vi "JIO_OnePannel_ChannelSweep_Ken.vi"() -> ()   [LabVIEW 2023, in "JIO.lvlib"]
uses:
  JIO.lvlib
  CTL/Mode_tx1_rx2.ctl
  FTDI/JIO/CLC_JIO_FTDI.lvlib
  R_S/R_S.lvlib
  Anritsu/Anritsu.lvlib
panel:
  in  "Mode":T1=enum."Tx"
  in  "ud att":i32
  in  "AvgTimes":i32=1
  in  "SA":refnum<visa-resource-name>="TCPIP0::192.168.100.202::inst0::INSTR"
  in  "File_note":string
  out "error out":errorcluster
  out "Time(64-Steps)sec":dbl
  out "Phase":i32
  out "Channel":i32
  out "IC_No.":i32
  out "Chain":i32
  out "Spectrum":dbl[](graph)
  in  "Waiting Time(ms)":u32=1000
  in  "error in":errorcluster
  in  "Ref_gain":i32
  in  "Ref_Phase":i32
  in  "Ref_Channel":i32
  in  "Ref_IC_":i32
  in  "Ref_Chain":i32
  in  "Channel_setting":T2
  # "CLC Gen4 8x4 Channel Sweep for TMYTEK"
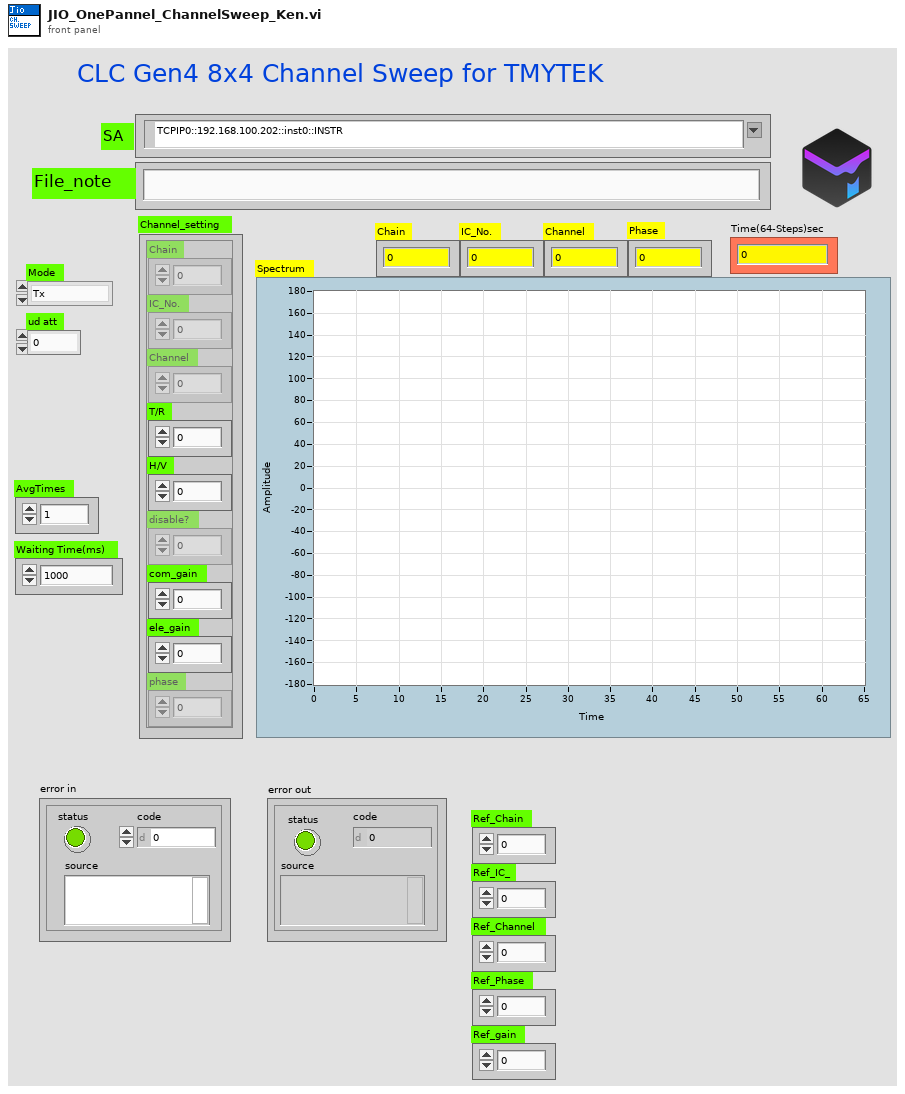
[diagram p1: front panel]
types:
  T1 = typedef "Mode_tx1_rx2.ctl" = enum16{"Standy", "Tx", "Rx"}
  T2 = cluster{"Chain":i32, "IC_No.":i32, "Channel":i32, "T/R":i32, "H/V":i32, "disable?":i32, "com_gain":i32, "ele_gain":i32, "phase":i32}
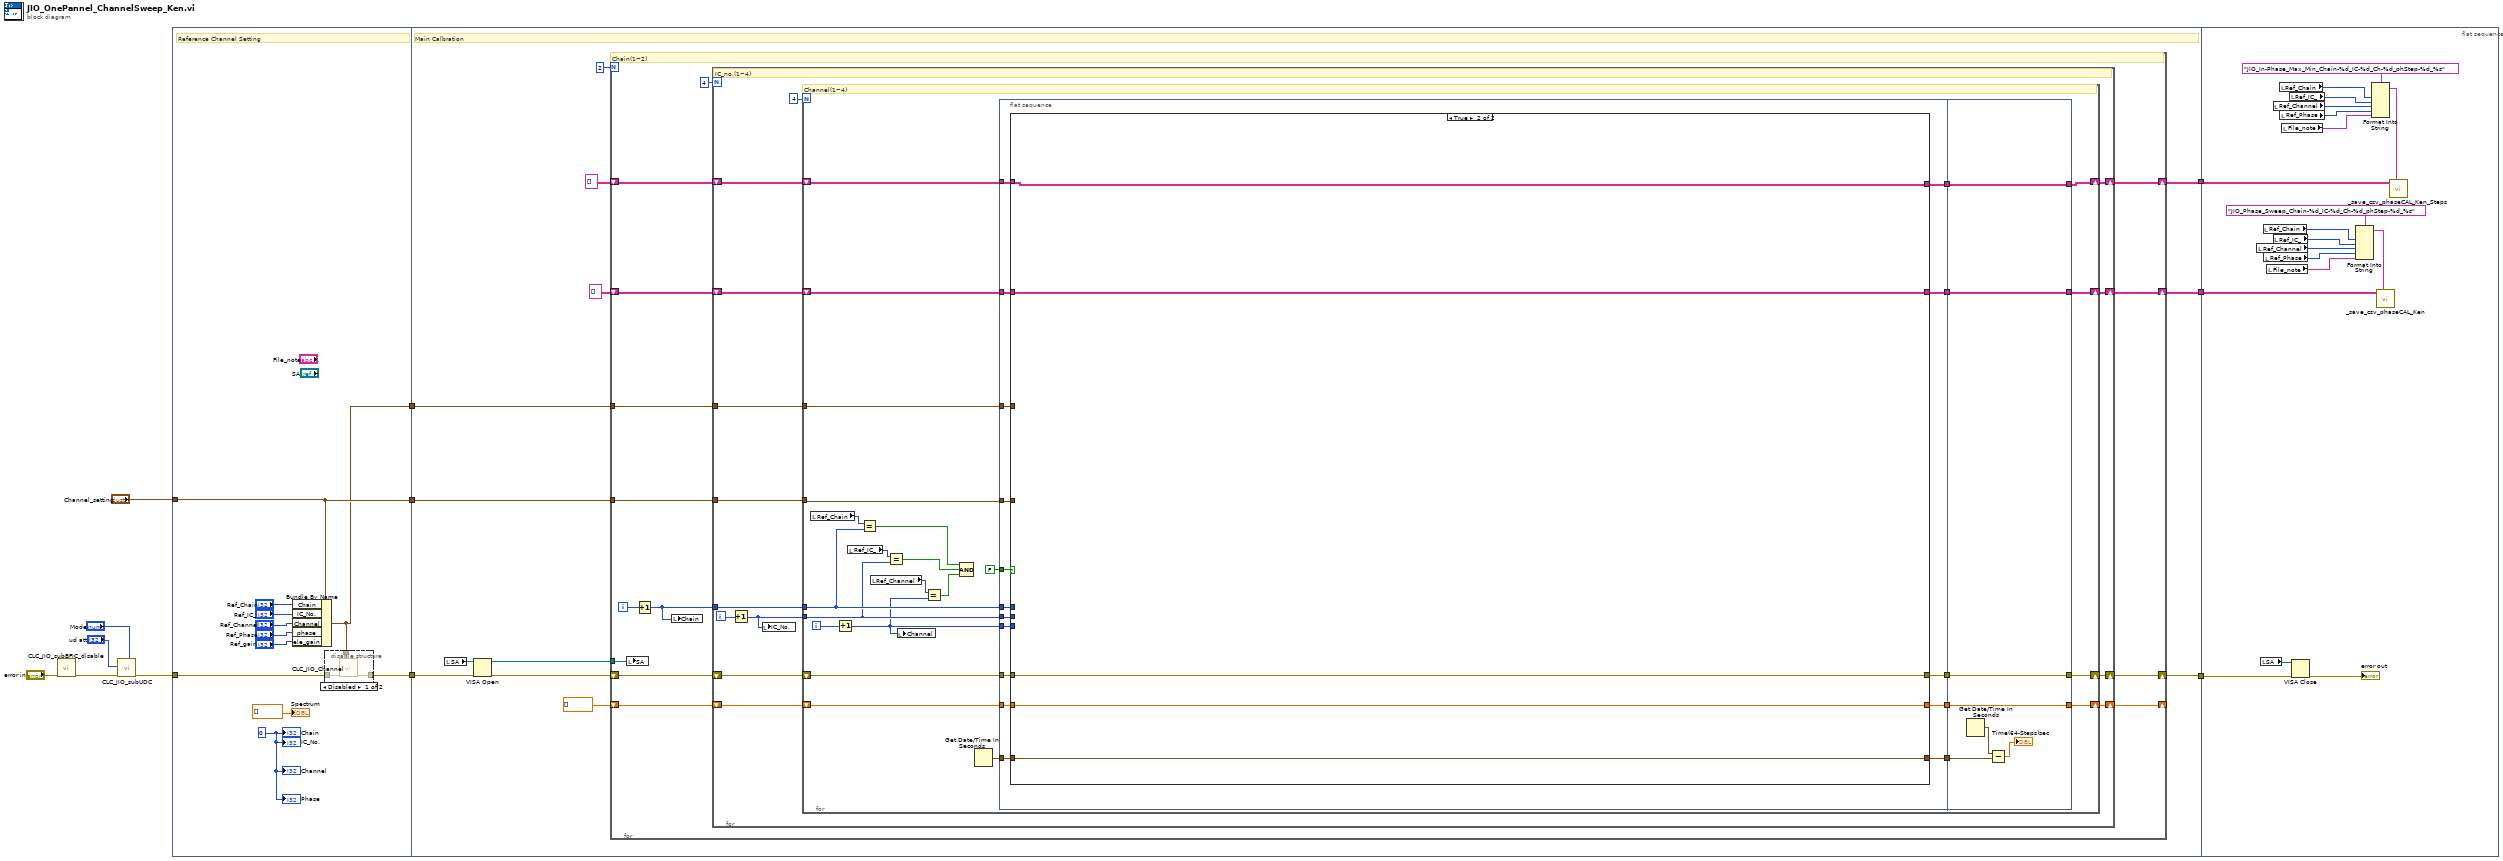
[diagram p0: block diagram]
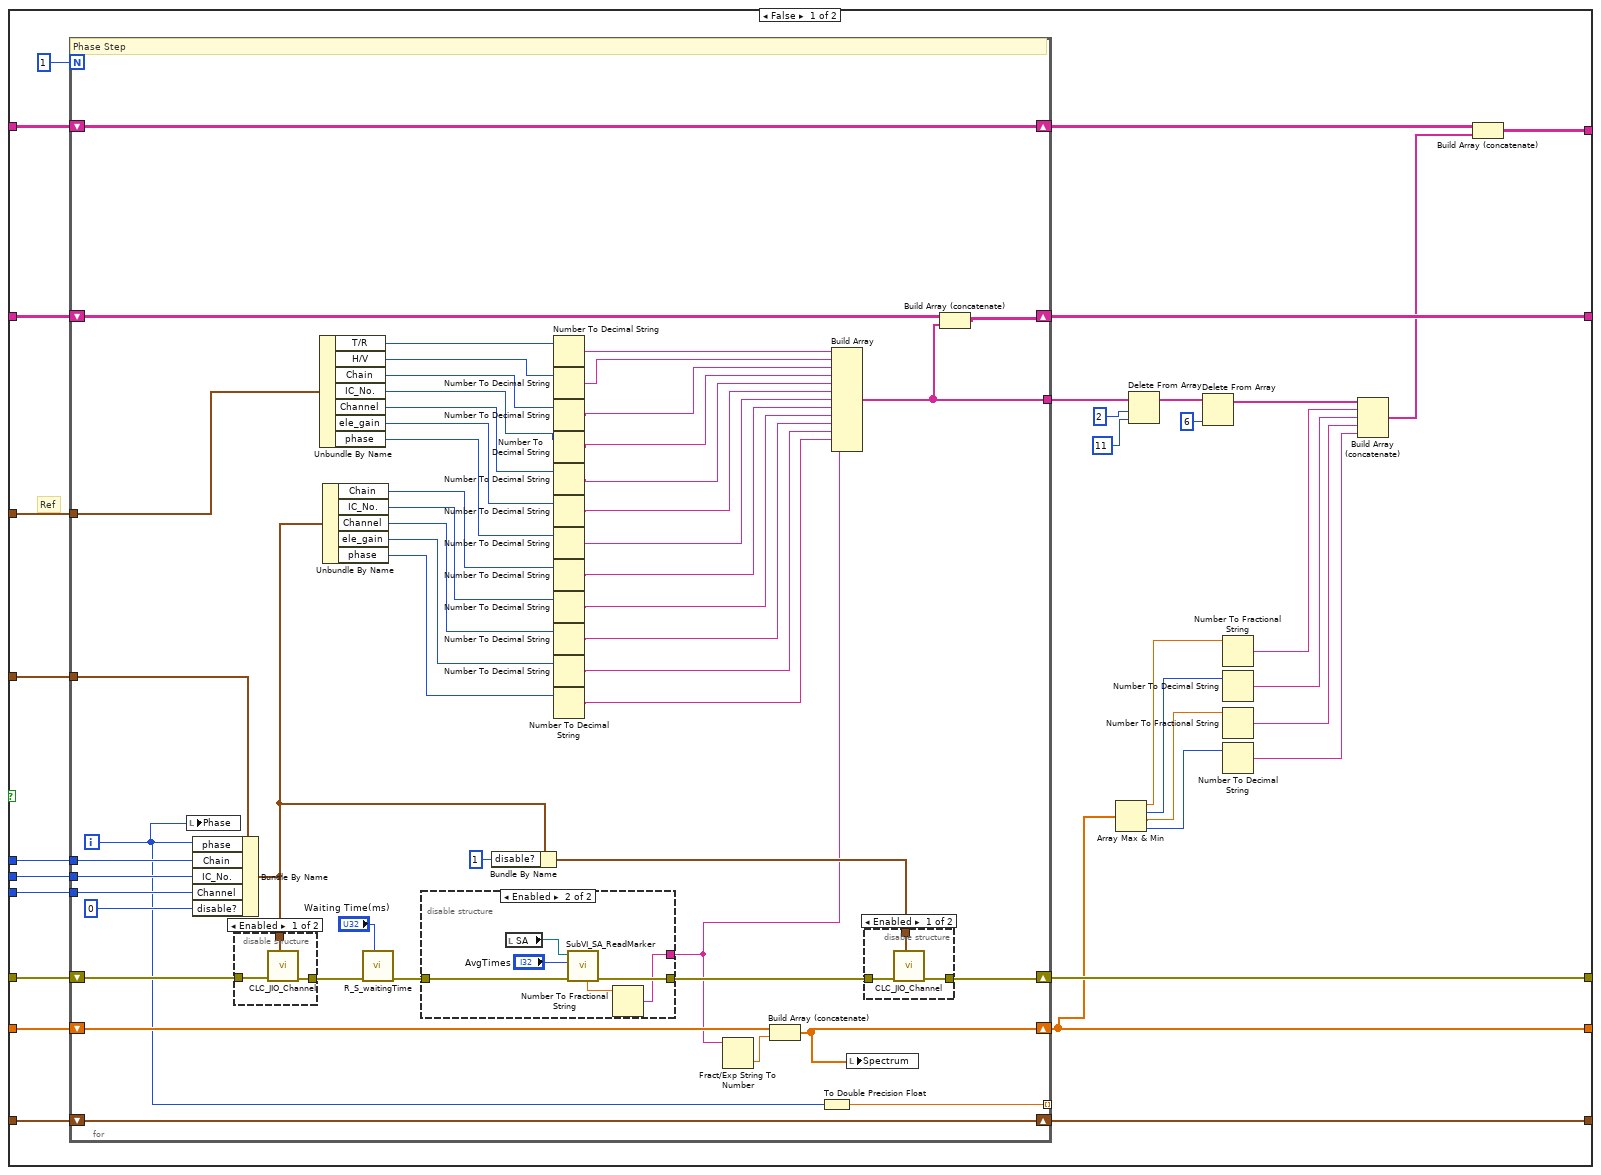
[diagram p3: hidden frame]
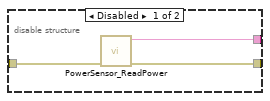
[diagram p4: hidden frame]
diagram:
  n1 = call "CLC_JIO_subBFIC_disable.vi"("error in"="error in") -> ("error out"=w4:errorcluster)  [unwired: 9 in, 1 out]
  n2 = call "CLC_JIO_subUDC.vi"("Mode"="Mode", "error in"=w4, "ud att"="ud att") -> ("error out"=w3:errorcluster)  [unwired: 7 in, 1 out]
  n3 = flat-sequence {
    tunnel: "Channel_setting" -> [w23]
    tunnel: [w23] -> w11
    tunnel: w3 -> [w17]
    tunnel: [w16] -> w10
    tunnel: [w13] -> w9
    tunnel: w11 -> [w39]
    tunnel: w10 -> [w31]
    tunnel: w9 -> [w38]
    tunnel: [w36] -> w8
    tunnel: [w35] -> w7
    tunnel: [w33] -> w6
    tunnel: w8 -> [w224]
    tunnel: w7 -> [w241]
    tunnel: w6 -> [w228]
    frame #0 {
      w14 = 0 ("Chain")
      # "Reference Channel Setting"
      n4 = Bundle By Name(cluster=w23, "Chain"="Ref_Chain", "IC_No."="Ref_IC_", "Channel"="Ref_Channel", "phase"="Ref_Phase", "ele_gain"="Ref_gain") -> (w13:T2)
      n5 = disable-structure shown="Disabled" {
        disable-tunnel: w17 -> [w26 w27]
        disable-tunnel: [w25 w27] -> w16
        disable-tunnel: w13 -> [w24 _]
        frame Disabled {
          n6 = call "CLC_JIO_Channel.vi"("Channel_setting"=w24, "error in"=w26) -> ("error out"=w25:errorcluster)  [unwired: 8 in, 1 out]
        }
        frame Enabled {
        }
      }
      "Spectrum" <- dbl[] [] ("Power Sensor (dB)")
      "Chain" <- w14
      "IC_No." <- w14
      "Channel" <- w14
      "Phase" <- w14
    }
    frame #1 {
      # "Main Calbration"
      n7 = local read "SA"() -> (w30:refnum<visa-resource-name>)
      n8 = VISA Open(error in (no error)=w31, VISA resource name=w30) -> (VISA resource name=w28:refnum<visa-resource-name>, error out=w32:errorcluster)  [unwired: 3 in]
      n9 = for {
        N: 2 -> [_]
        tunnel: w39 -> [w53]
        shift-right: [w51] -> w36
        shift-left: w32 -> [w52]
        tunnel: w38 -> [w49]
        shift-right: [w47] -> w35
        shift-left: string[][] [] -> [w48]
        shift-right: [w45] -> w33
        shift-left: string[][] [] -> [w46]
        shift-right: [w42] -> _
        shift-left: dbl[] [] ("Power Sensor (dB)") -> [w43]
        tunnel: w28 -> [w41]
        i -> [w50]
        # "Chain(1~2)"
        n10 = local write "SA"(w41) -> ()
        n11 = Increment(x=w50) -> (x+1=w44:i32)
        n12 = local write "Chain"(w44) -> ()
        n13 = for {
          N: 4 -> [_]
          tunnel: w53 -> [w67]
          tunnel: w44 -> [w66]
          shift-right: [w64] -> w51
          shift-left: w52 -> [w65]
          tunnel: w49 -> [w62]
          shift-right: [w60] -> w47
          shift-left: w48 -> [w61]
          shift-right: [w58] -> w45
          shift-left: w46 -> [w59]
          shift-right: [w55] -> w42
          shift-left: w43 -> [w56]
          i -> [w63]
          # "IC_no.(1~4)"
          n14 = Increment(x=w63) -> (x+1=w57:i32)
          n15 = local write "IC_No."(w57) -> ()
          n16 = for {
            N: 4 -> [_]
            tunnel: w67 -> [w94]
            tunnel: w57 -> [w74]
            tunnel: w66 -> [w75]
            shift-right: [w87] -> w64
            shift-left: w65 -> [w95]
            tunnel: w62 -> [w85]
            shift-right: [w83] -> w60
            shift-left: w61 -> [w84]
            shift-right: [w76] -> w58
            shift-left: w59 -> [w78]
            shift-right: [w71] -> w55
            shift-left: w56 -> [w72]
            i -> [w86]
            # "Channel(1~4)"
            n17 = local read "Ref_Chain"() -> (w93:i32)
            n18 = Increment(x=w86) -> (x+1=w73:i32)
            n19 = local read "Ref_IC_"() -> (w92:i32)
            n20 = Equal?(x=w93, y=w75) -> (x = y?=w90:bool)
            n21 = local read "Ref_Channel"() -> (w91:i32)
            n22 = Equal?(x=w92, y=w74) -> (x = y?=w89:bool)
            n23 = local write "Channel"(w73) -> ()
            n24 = Equal?(x=w91, y=w73) -> (x = y?=w88:bool)
            n25 = Compound Arithmetic op=AND(w90, w89, w88) -> ()  [unwired: 1 out]
            n26 = Get Date/Time In Seconds() -> (seconds since 1Jan1904=w82:timestamp)
            n27 = flat-sequence {
              tunnel: w95 -> [w111]
              tunnel: w94 -> [w110]
              tunnel: w75 -> [w109]
              tunnel: w74 -> [w108]
              tunnel: FALSE -> [w107]
              tunnel: w72 -> [w106]
              tunnel: w73 -> [w104]
              tunnel: w85 -> [w103]
              tunnel: w84 -> [w102]
              tunnel: w82 -> [w100]
              tunnel: [w105] -> w81
              tunnel: [w101] -> w80
              tunnel: [w99] -> w79
              tunnel: w78 -> [w98]
              tunnel: [w97] -> w77
              tunnel: [w96] -> w70
              tunnel: [w221] -> w83
              tunnel: [w222] -> w87
              tunnel: w81 -> [w222]
              tunnel: w80 -> [w221]
              tunnel: w79 -> [w218]
              tunnel: w77 -> [w217]
              tunnel: [w217] -> w76
              tunnel: [w216] -> w71
              tunnel: w70 -> [w216]
              frame #0 {
                n28 = case shown="True" w107 {
                  tunnel: w109 -> [w143 _]
                  tunnel: w108 -> [w142 _]
                  tunnel: w104 -> [w141 _]
                  tunnel: w111 -> [w140 w215]
                  tunnel: w110 -> [w139 _]
                  tunnel: [w137 w215] -> w105
                  tunnel: w106 -> [w136 w211]
                  tunnel: w103 -> [w135 _]
                  tunnel: w102 -> [w134 w214]
                  tunnel: [w133 w214] -> w101
                  tunnel: w100 -> [w132 w213]
                  tunnel: [w131 w213] -> w99
                  tunnel: w98 -> [w116 w212]
                  tunnel: [w113 w212] -> w97
                  tunnel: [w112 w211] -> w96
                  frame False {
                    # "Ref"
                    n29 = for {
                      N: 1 -> [_]
                      tunnel: w143 -> [w193]
                      tunnel: w142 -> [w192]
                      tunnel: w141 -> [w191]
                      tunnel: w139 -> [w177]
                      shift-right: [w184] -> w137
                      shift-left: w140 -> [w190]
                      shift-right: [w179] -> w112
                      shift-left: w136 -> [w181]
                      tunnel: w135 -> [w173]
                      shift-right: [w151] -> w133
                      shift-left: w134 -> [w150]
                      shift-right: [w148] -> w131
                      shift-left: w132 -> [w148]
                      tunnel: [w146] -> _ mode=indexing
                      tunnel: [w145] -> w130
                      shift-right: [w144] -> w115
                      shift-left: w116 -> [w144]
                      i -> [w147]
                      # "Phase Step"
                      n30 = local write "Phase"(w147) -> ()
                      n31 = Bundle By Name(cluster=w177, "phase"=w147, "Chain"=w193, "IC_No."=w192, "Channel"=w191, "disable?"=0) -> (w178:T2)
                      n32 = disable-structure shown="Enabled" {
                        disable-tunnel: w190 -> [w209 w210]
                        disable-tunnel: [w208 w210] -> w188
                        disable-tunnel: w178 -> [w207 _]
                        frame Enabled {
                          n33 = call "CLC_JIO_Channel.vi"("Channel_setting"=w207, "error in"=w209) -> ("error out"=w208:errorcluster)  [unwired: 8 in, 1 out]
                        }
                        frame Disabled {
                        }
                      }
                      n34 = Unbundle By Name(w173) -> ("T/R"=w176:i32, "H/V"=w175:i32, "Chain"=w174:i32, "IC_No."=w172:i32, "Channel"=w171:i32, "ele_gain"=w170:i32, "phase"=w169:i32)
                      n35 = Unbundle By Name(w178) -> ("Chain"=w168:i32, "IC_No."=w167:i32, "Channel"=w166:i32, "ele_gain"=w165:i32, "phase"=w164:i32)
                      n36 = call "R_S_waitingTime.vi"("Waiting Time(ms)"="Waiting Time(ms)", "error in"=w188) -> ("error out"=w183:errorcluster)  [unwired: 9 in]
                      n37 = disable-structure shown="Enabled" {
                        disable-tunnel: w183 -> [w196 w202]
                        disable-tunnel: [w195 w201] -> w182
                        disable-tunnel: [w194 w198] -> w149
                        frame Disabled {
                          n38 = call "PowerSensor_ReadPower.vi"("error in"=w196) -> ("error out"=w195:errorcluster, "Response"=w194:string)  [unwired: 9 in]
                        }
                        frame Enabled {
                          n39 = local read "SA"() -> (w197:refnum<visa-resource-name>)
                          n40 = call "SubVI_SA_ReadMarker.vi"("error in (no error)"=w202, "AvgTimes"="AvgTimes", "VISA resource name"=w197) -> ("error out"=w201:errorcluster, "Marker Power"=w199:dbl)  [unwired: 5 in, 2 out]
                          n41 = Number To Fractional String(number=w199) -> (F-format string=w198:string)  [unwired: 3 in]
                        }
                      }
                      n42 = Bundle By Name(cluster=w178, "disable?"=1) -> (w185:T2)
                      n43 = Number To Decimal String(number=w176) -> (decimal integer string=w163:string)  [unwired: 1 in]
                      n44 = Number To Decimal String(number=w175) -> (decimal integer string=w162:string)  [unwired: 1 in]
                      n45 = Number To Decimal String(number=w174) -> (decimal integer string=w161:string)  [unwired: 1 in]
                      n46 = Number To Decimal String(number=w172) -> (decimal integer string=w160:string)  [unwired: 1 in]
                      n47 = Number To Decimal String(number=w171) -> (decimal integer string=w159:string)  [unwired: 1 in]
                      n48 = Number To Decimal String(number=w170) -> (decimal integer string=w158:string)  [unwired: 1 in]
                      n49 = Number To Decimal String(number=w169) -> (decimal integer string=w157:string)  [unwired: 1 in]
                      n50 = Number To Decimal String(number=w168) -> (decimal integer string=w156:string)  [unwired: 1 in]
                      n51 = Number To Decimal String(number=w167) -> (decimal integer string=w155:string)  [unwired: 1 in]
                      n52 = Number To Decimal String(number=w166) -> (decimal integer string=w154:string)  [unwired: 1 in]
                      n53 = Number To Decimal String(number=w165) -> (decimal integer string=w153:string)  [unwired: 1 in]
                      n54 = Number To Decimal String(number=w164) -> (decimal integer string=w152:string)  [unwired: 1 in]
                      n55 = Fract/Exp String To Number(string=w149) -> (number=w180:dbl)  [unwired: 3 in, 1 out]
                      n56 = Build Array (concatenate)(w181, w180) -> (w179:dbl[])
                      n57 = To Double Precision Float(number=w147) -> (double precision float=w146:dbl)
                      n58 = Build Array(w163, w162, w161, w160, w159, w158, w157, w156, w155, w154, w153, w152, w149) -> (w145:string[])
                      n59 = local write "Spectrum"(w179) -> ()
                      n60 = disable-structure shown="Enabled" {
                        disable-tunnel: w185 -> [w205 _]
                        disable-tunnel: [w204 w206] -> w184
                        disable-tunnel: w182 -> [w203 w206]
                        frame Enabled {
                          n61 = call "CLC_JIO_Channel.vi"("Channel_setting"=w205, "error in"=w203) -> ("error out"=w204:errorcluster)  [unwired: 8 in, 1 out]
                        }
                        frame Disabled {
                        }
                      }
                      n62 = Build Array (concatenate)(w150, w145) -> (w151:string[][])
                    }
                    n63 = Array Max & Min(array=w112) -> (max value=w124:dbl, max index (indices)=w122:i32, min value=w121:dbl, min index (indices)=w120:i32)
                    n64 = Delete From Array(array=w130, length=2, index=11) -> (array with subset deleted=w127:string[])  [unwired: 1 out]
                    n65 = Delete From Array(array=w127, index=6) -> (array with subset deleted=w125:string[])  [unwired: 1 in, 1 out]
                    n66 = Number To Fractional String(number=w124) -> (F-format string=w123:string)  [unwired: 3 in]
                    n67 = Number To Decimal String(number=w122) -> (decimal integer string=w119:string)  [unwired: 1 in]
                    n68 = Number To Fractional String(number=w121) -> (F-format string=w118:string)  [unwired: 3 in]
                    n69 = Number To Decimal String(number=w120) -> (decimal integer string=w117:string)  [unwired: 1 in]
                    n70 = Build Array (concatenate)(w125, w123, w119, w118, w117) -> (w114:string[])
                    n71 = Build Array (concatenate)(w115, w114) -> (w113:string[][])
                  }
                  frame True {
                  }
                }
              }
              frame #1 {
                n72 = Get Date/Time In Seconds() -> (seconds since 1Jan1904=w219:timestamp)
                n73 = Subtract(x=w219, y=w218) -> (x-y=→"Time(64-Steps)sec":dbl)
              }
            }
          }
        }
      }
    }
    frame #2 {
      n74 = local read "Ref_Channel"() -> (w236:i32)
      n75 = local read "SA"() -> (w223:refnum<visa-resource-name>)
      n76 = local read "Ref_Chain"() -> (w238:i32)
      n77 = local read "Ref_Phase"() -> (w235:i32)
      n78 = local read "File_note"() -> (w227:string)
      n79 = local read "Ref_Channel"() -> (w233:i32)
      n80 = local read "Ref_IC_"() -> (w237:i32)
      n81 = local read "Ref_Chain"() -> (w231:i32)
      n82 = local read "Ref_Phase"() -> (w234:i32)
      n83 = local read "File_note"() -> (w226:string)
      n84 = local read "Ref_IC_"() -> (w232:i32)
      n85 = VISA Close(VISA resource name=w223, error in (no error)=w224) -> (error out=→"error out":errorcluster)
      n86 = Format Into String(format string="JIO_Phase_Sweep_Chain-%d_IC-%d_Ch-%d_phStep-%d_%s", w238, w237, w236, w235, w227) -> (resulting string=w239:string)  [unwired: 2 in, 1 out]
      n87 = Format Into String(format string="JIO_In-Phase_Max_Min_Chain-%d_IC-%d_Ch-%d_phStep-%d_%s", w231, w232, w233, w234, w226) -> (resulting string=w230:string)  [unwired: 2 in, 1 out]
      n88 = call "_save_csv_phaseCAL_Ken.vi"("NoteName"=w239, "array in"=w241) -> ()  [unwired: 10 in]
      n89 = call "_save_csv_phaseCAL_Ken_Steps.vi"("NoteName"=w230, "array in"=w228) -> ()  [unwired: 10 in]
    }
  }
